vi "Constants.vi"() -> ()   [LabVIEW 2014, in "UEGO Sim Shared.lvlib"]
doc: "Use this Global VI to access the GUIDs assigned to the page resources of the Custom Device."
uses:
  UEGO Sim Shared.lvlib
panel:
  in  "Tab Control":enum32{"GUIDS", "Constants", "Properties"}(tab)
  in  "Page 5":string="eff91030-b094-432c-86b5-e9f9502e4693"
  in  "Page 4":string="2502f0ca-0aba-45b5-b01b-0f7b7f0c4a8c"
  in  "Page 3":string="afc96efb-b967-4bef-868c-082550866938"
  in  "Page 2":string="569ccfd6-fa64-42dd-911f-acb180f9186f"
  in  "Page 1":string="d13521bb-97e5-484c-a1b4-8ffd303a4e5e"
  in  "UEGO Sim":string="ff7a9f46-4f61-4499-baf7-cd41c676dfd4"
  in  "thermal model rate":dbl=100.0
  in  "RIO target":string="RIO0"
  in  "ambient exhaust temp":dbl=100.0
  in  "heat param c":dbl=960.0
  in  "heat param b":dbl=40.0
  in  "heat param a":dbl=55000.0
  in  "params.bitfile":string="bitfile"
  in  "params.heat param a":string="heat param a"
  in  "params.heat param b":string="heat param b"
  in  "params.heat param c":string="heat param c"
  in  "params.ambient exhaust temp":string="ambient exhaust temp"
  in  "params.RIO target":string="rio target"
  in  "params.thermal model rate":string="thermal model rate"
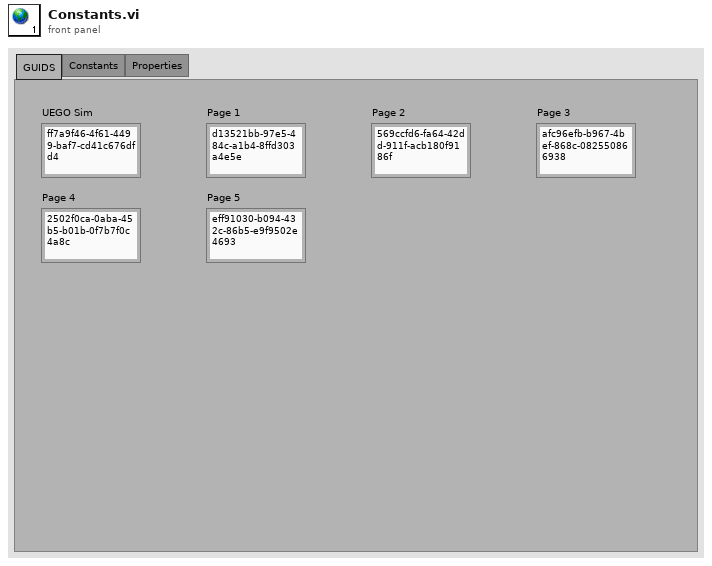
[diagram p1: front panel]
diagram:
